vi "Write yCorrection_arcsec.vi"(8 "error in (no error)":errorcluster, 10 "yCorrection_arcsec":dbl[unit] min=-0.001454441043328608 max=0.001454441043328608, 11 "AOSPointingOffset in":refnum<class "AOSPointingOffset.lvclass">) -> (0 "error out":errorcluster, 3 "AOSPointingOffset out":refnum<class "AOSPointingOffset.lvclass">)   [LabVIEW 2022 SP3, in "TCSDataDefinitions.lvlib" / "TCSActiveOpticsCommand.lvlib" / "AOSPointingOffset.lvclass"]
uses:
  AOSPointingOffset.lvclass
  AOSPointingOffset.lvclass/AOSPointingOffset.ctl
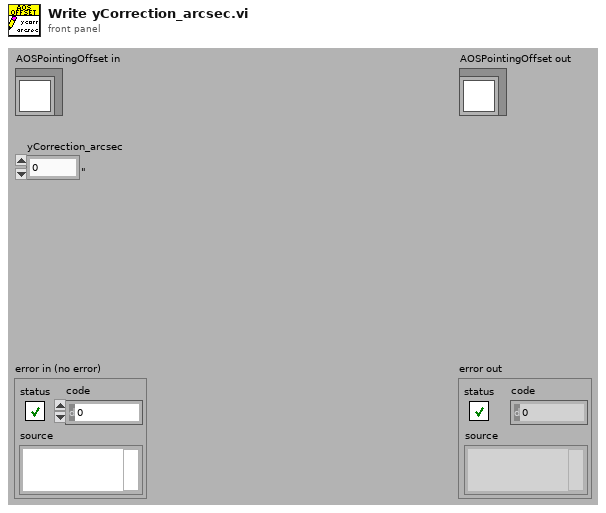
[diagram p1: front panel]
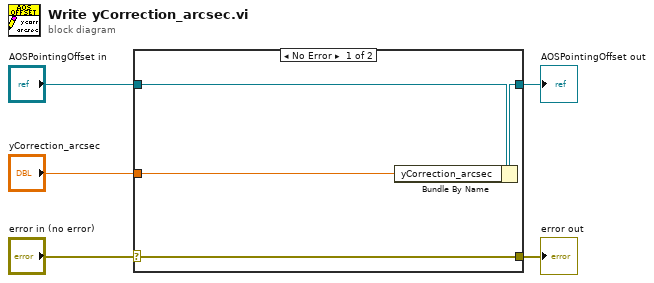
[diagram p0: block diagram]
diagram:
  n1 = case shown="No Error" "error in (no error)" {
    selector: "error in (no error)" -> [w9 w10]
    tunnel: [w9 w10] -> w4
    tunnel: [w7 w11] -> w2
    tunnel: "AOSPointingOffset in" -> [w8 w11]
    tunnel: "yCorrection_arcsec" -> [w6 _]
    frame No Error {
      n2 = Bundle By Name(cluster=w8, "yCorrection_arcsec"=w6) -> (w7:refnum<class "AOSPointingOffset.lvclass">)
    }
    frame Error {
    }
  }
  "error out" <- w4
  "AOSPointingOffset out" <- w2
